vi "State Logic.vi"(10 "Level":dbl, 11 "Level Controller in":refnum<class "Level Controller.lvclass">) -> (1 "State Changed":bool, 2 "Output State":bool, 3 "Level Controller out":refnum<class "Level Controller.lvclass">)   [LabVIEW 2012, in "Level Controller.lvlib" / "Level Controller.lvclass"]
uses:
  Level Controller.lvclass
  Level Controller.lvclass/Level Controller.ctl
  Value Position.ctl
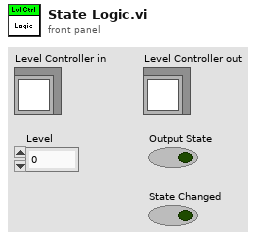
[diagram p1: front panel]
types:
  T1 = typedef "Level Controller.lvlib/Level Controller.lvclass/Value Position.ctl" = enum16{"Never Assigned", "Above Level", "Below Level"}
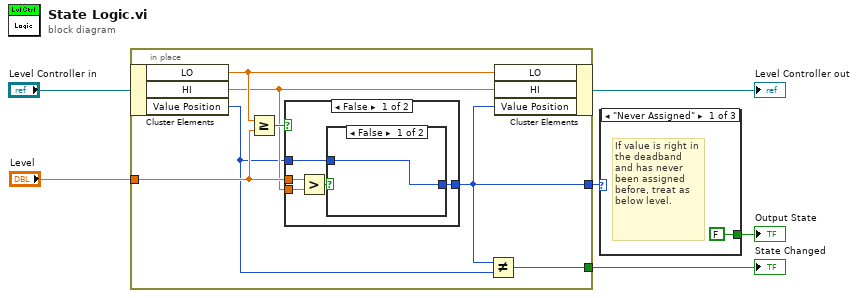
[diagram p0: block diagram]
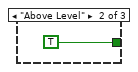
[diagram p2: hidden frame]
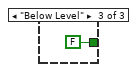
[diagram p3: hidden frame]
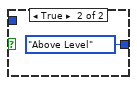
[diagram p4: hidden frame]
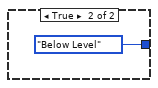
[diagram p5: hidden frame]
diagram:
  n1 = in-place {
    in-place-border: "Level" -> [w11]
    in-place-border: [w13] -> w4
    in-place-border: [w8] -> w5
    n2 = in-place-cluster #1("Level Controller in") -> ("LO"=w12:dbl, "HI"=w9:dbl, "Value Position"=w7:T1)
    n3 = Greater Or Equal?(x=w12, y=w11) -> (x >= y?=w10:bool)
    n4 = case shown="False" w10 {
      tunnel: w11 -> [w18 _]
      tunnel: [w16 Value_Position."Below Level" ("Deadband.Value Position")] -> w8
      tunnel: w9 -> [w17 _]
      tunnel: w7 -> [w14 _]
      frame False {
        n5 = Greater?(x=w18, y=w17) -> (0:w15:bool)
        n6 = case shown="False" w15 {
          tunnel: [w19 Value_Position."Above Level" ("Deadband.Value Position")] -> w16
          tunnel: w14 -> [w19 _]
          frame False {
          }
          frame True {
          }
        }
      }
      frame True {
      }
    }
    n7 = Not Equal?(x=w8, y=w7) -> (x != y?=w13:bool)
    n8 = in-place-cluster #1("LO"=w12, "HI"=w9, "Value Position"=w8) -> (→"Level Controller out":refnum<class "Level Controller.lvclass">)
  }
  "State Changed" <- w4
  n9 = case shown="\"Never Assigned\"" w5 {
    tunnel: [FALSE TRUE FALSE] -> w6
    frame "Never Assigned" {
      # "If value is right in the deadband and has never been assigned before, treat as below level."
    }
    frame "Above Level" {
    }
    frame "Below Level" {
    }
  }
  "Output State" <- w6
